vi "Analys DOWN.vi"(8 "error in":errorcluster, 11 "data":T1) -> (0 "error out":errorcluster, 2 "output cluster":cluster{"Array":dbl[], "Array":dbl[]})   [LabVIEW 2019]
uses:
  Interrogator/Analys Argument--cluster.ctl
  TypeDef/Analys data.ctl
  TypeDef/Analys type.ctl
  TypeDef/Sett data.ctl
  TypeDef/ISO.ctl
  TypeDef/Noise.ctl
  TypeDef/Link.ctl
  Class/ISO 14443 A DOWN.lvclass
  Class/ISO 14443 B DOWN.lvclass
  Class/Felica DOWN.lvclass
  Class/ISO 15693 DOWN.lvclass
  Interrogator/DOWNLINK.lvlib
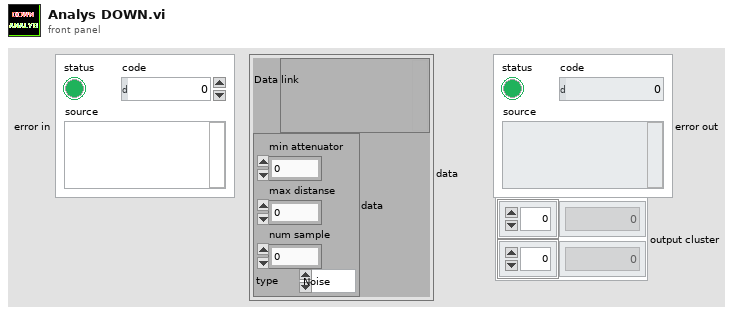
[diagram p1: front panel]
types:
  T1 = typedef "DOWNLINK.lvlib/Analys Argument--cluster.ctl" = cluster{"Data link":variant, "data":T2}
  T2 = typedef "Analys data.ctl" = cluster{"min attenuator":dbl, "max distanse":dbl, "num sample":dbl, "type":T3}
  T3 = typedef "Analys type.ctl" = enum16{"Noise", "Distance"}
  T4 = typedef "Sett data.ctl" = cluster{"Filter":i32, "Gain":dbl, "Bit rate":dbl, "ISO/IEC w ":T5, "BI":cluster{"R":dbl, "C":dbl, "L":dbl}, "BM":cluster{"R":dbl, "C":dbl, "L":dbl}, "M":cluster{"Метка":i64, "Считыветель":i64}, "Type noise":T6, "Link":T7, "Noise attenuator":dbl, "Signal gain":dbl, "Distance":dbl}
  T5 = typedef "ISO.ctl" = enum16{"14443 Type A", "14443 Type B", "Felica", "15693"}
  T6 = typedef "Noise.ctl" = enum16{"Гауссовский шум", "Белый шум"}
  T7 = typedef "Link.ctl" = enum16{"UPLINK", "DOWNLINK"}
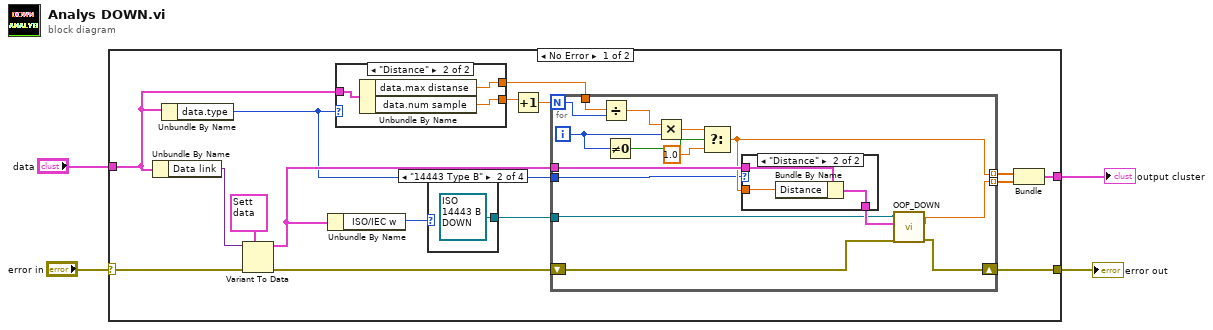
[diagram p0: block diagram]
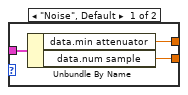
[diagram p2: hidden frame]
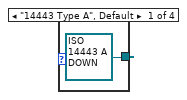
[diagram p3: hidden frame]
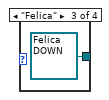
[diagram p4: hidden frame]
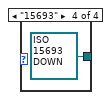
[diagram p5: hidden frame]
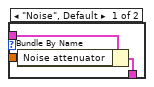
[diagram p6: hidden frame]
diagram:
  n1 = case shown="No Error" "error in" {
    selector: "error in" -> [w14 w52]
    tunnel: [w16 w52] -> w4
    tunnel: "data" -> [w6 _]
    tunnel: [w10 _] -> w2
    frame No Error {
      n2 = Unbundle By Name(w6) -> ("Data link"=w20:variant)
      n3 = Unbundle By Name(w6) -> ("data.type"=w5:T3)
      n4 = Variant To Data(error in=w14, type=T4 {"Filter"=0, "Gain"=0.0, "Bit rate"=0.0, "ISO/IEC w "=enum."14443 Type A", "BI"={"R"=0.0, "C"=0.0, "L"=0.0}, "BM"={"R"=0.0, "C"=0.0, "L"=0.0}, "M"={"Метка"=4, "Считыветель"=4}, "Type noise"=enum."Гауссовский шум", "Link"=enum."UPLINK", "Noise attenuator"=0.0, "Signal gain"=1.0, "Distance"=0.0} ("Sett data"), Variant=w20) -> (data=w15:T4, error out=w17:errorcluster)
      n5 = Unbundle By Name(w15) -> ("ISO/IEC w"=w9:T5)
      n6 = case shown="\"Distance\"" w5 {
        tunnel: [w23 w24] -> w18
        tunnel: w6 -> [w22 w26]
        tunnel: [w21 w25] -> w13
        frame "Noise", Default {
          n7 = Unbundle By Name(w22) -> ("data.min attenuator"=w21:dbl, "data.num sample"=w23:dbl)
        }
        frame "Distance" {
          n8 = Unbundle By Name(w26) -> ("data.max distanse"=w25:dbl, "data.num sample"=w24:dbl)
        }
      }
      n9 = case shown="\"14443 Type B\"" w9 {
        tunnel: [refnum<class "ISO 14443 A DOWN.lvclass"> refnum ("ISO 14443 A DOWN.lvclass") refnum<class "ISO 14443 B DOWN.lvclass"> refnum ("ISO 14443 B DOWN.lvclass") refnum<class "Felica DOWN.lvclass"> refnum ("Felica DOWN.lvclass") refnum<class "ISO 15693 DOWN.lvclass"> refnum ("ISO 15693 DOWN.lvclass")] -> w8
        frame "14443 Type A", Default {
        }
        frame "14443 Type B" {
        }
        frame "Felica" {
        }
        frame "15693" {
        }
      }
      n10 = Increment(x=w18) -> (x+1=w7:dbl)
      n11 = for {
        N: w7 -> [w45]
        shift-right: [w40] -> w16
        shift-left: w17 -> [w41]
        tunnel: w8 -> [w37]
        tunnel: w15 -> [w43]
        tunnel: [w32] -> w12 mode=indexing
        tunnel: [w39] -> w11 mode=indexing
        tunnel: w13 -> [w42]
        tunnel: w5 -> [w31]
        i -> [w35]
        n12 = Divide(x=w42, y=w45) -> (x/y=w44:dbl)
        n13 = Not Equal To 0?(x=w35) -> (x != 0?=w36:bool)
        n14 = Multiply(x=w44, y=w35) -> (x*y=w33:dbl)
        n15 = Select(t=w33, s=w36, f=1.0) -> (s? t:f=w32:dbl)
        n16 = case shown="\"Distance\"" w31 {
          tunnel: w43 -> [w48 w51]
          tunnel: [w47 w50] -> w38
          tunnel: w32 -> [w46 w49]
          frame "Noise", Default {
            n17 = Bundle By Name(cluster=w48, "Noise attenuator"=w46) -> (w47:T4)
          }
          frame "Distance" {
            n18 = Bundle By Name(cluster=w51, "Distance"=w49) -> (w50:T4)
          }
        }
        n19 = call "OOP_DOWN.vi"("error in (no error)"=w41, "Sett data"=w38, "RFID system.lvclass"=w37) -> ("error out"=w40:errorcluster, "Error on  byte"=w39:dbl)  [unwired: 5 in, 2 out]
      }
      n20 = Bundle(w12, w11) -> (w10:cluster{dbl[], dbl[]})  [unwired: 1 in]
    }
    frame Error {
    }
  }
  "error out" <- w4
  "output cluster" <- w2
